vi "Measurement UI.vi"() -> ()   [LabVIEW 2025, in "Example Plugin UI.lvlib"]
uses:
  Example Plugin UI.lvlib
  ExamplePluginOOBService_client/RPC Messages/hwval_BoolRequest.ctl
  ExamplePluginOOBService_client/RPC Messages/hwval_ExportRequest.ctl
  ExamplePluginOOBService_client/ExamplePluginOOBService_client.lvlib
panel:
  out "Export out":string
  out "PauseResume out":bool
  in  "Export File Type":string(combo)="RAW"
  in  "Export":bool
  in  "PauseResume":bool caption="Pause"
  out "OOB Port":i32
  out "string 2D array out":string[][](array[string])
  in  "string 2D array in":string[][](array[string])
  out "double 2D array out":dbl[][](array[numeric])
  in  "double 2D array in":dbl[][](array[numeric])
  out "xy data out":cluster{"x_data":dbl[], "y_data":dbl[]}(graph)
  out "u32 animal enum out":enum32{"Rabbit", "Gopher", "Badger"}(ring)=enum."Badger"
  out "u32 color ring out":u32(ring)=2 items=["Red", "Green", "Blue"]
  out "string out":string="Empty"
  out "bool out":bool
  out "I64 out":i64
  out "I64 array out":i64[](array[numeric])
  out "I32 out":i32
  out "I32 array out":i32[](array[numeric])
  out "U64 out":u64
  out "U64 array out":u64[](array[numeric])
  out "U32 out":u32
  out "U32 array out":u32[](array[numeric])
  out "double out":dbl
  out "double array out":dbl[](array[numeric])
  in  "u32 animal enum in":enum32{"Rabbit", "Gopher", "Badger"}(ring)
  in  "u32 color ring in":u32(ring) items=["Red", "Green", "Blue"]
  in  "string in":string
  in  "bool in":bool
  in  "I64 in":i64
  in  "I64 array in":i64[](array[numeric])
  in  "I32 in":i32
  in  "I32 array in":i32[](array[numeric])
  in  "U64 in":u64
  in  "U64 array in":u64[](array[numeric])
  in  "U32 in":u32
  in  "U32 array in":u32[](array[numeric])
  in  "double in":dbl
  in  "double array in":dbl[](array[numeric])
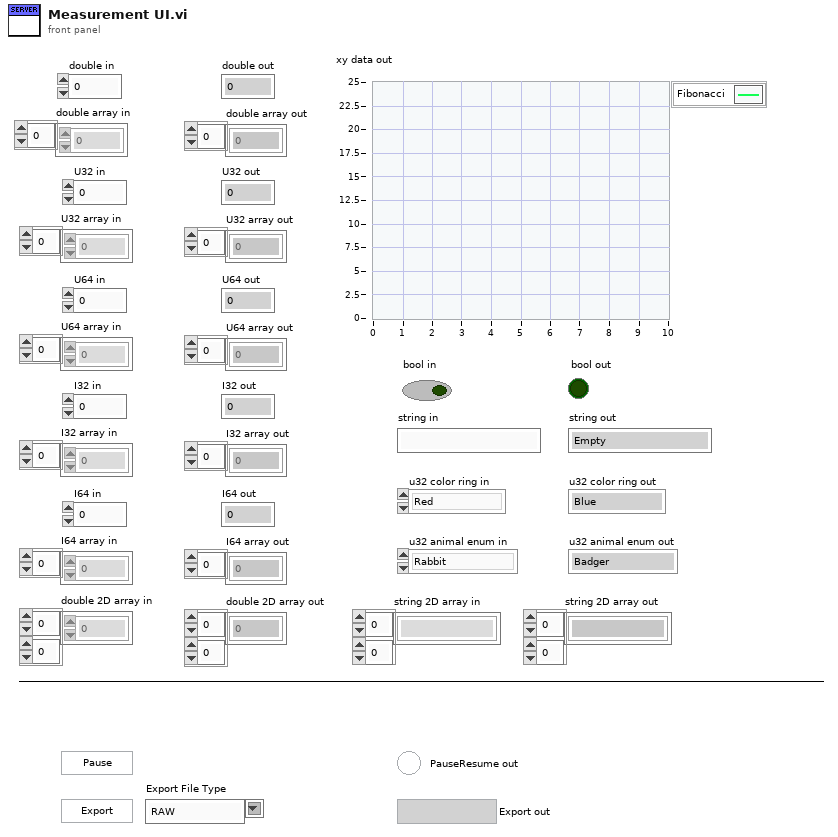
[diagram p1: front panel]
types:
  T1 = typedef "grpc-lvsupport-release.lvlib/grpcId.ctl" = u64
  T2 = typedef "ExamplePluginOOBService_client.lvlib/hwval_BoolRequest.ctl" = cluster{"BooleanData":bool}
  T3 = typedef "ExamplePluginOOBService_client.lvlib/hwval_ExportRequest.ctl" = cluster{"FileType":string}
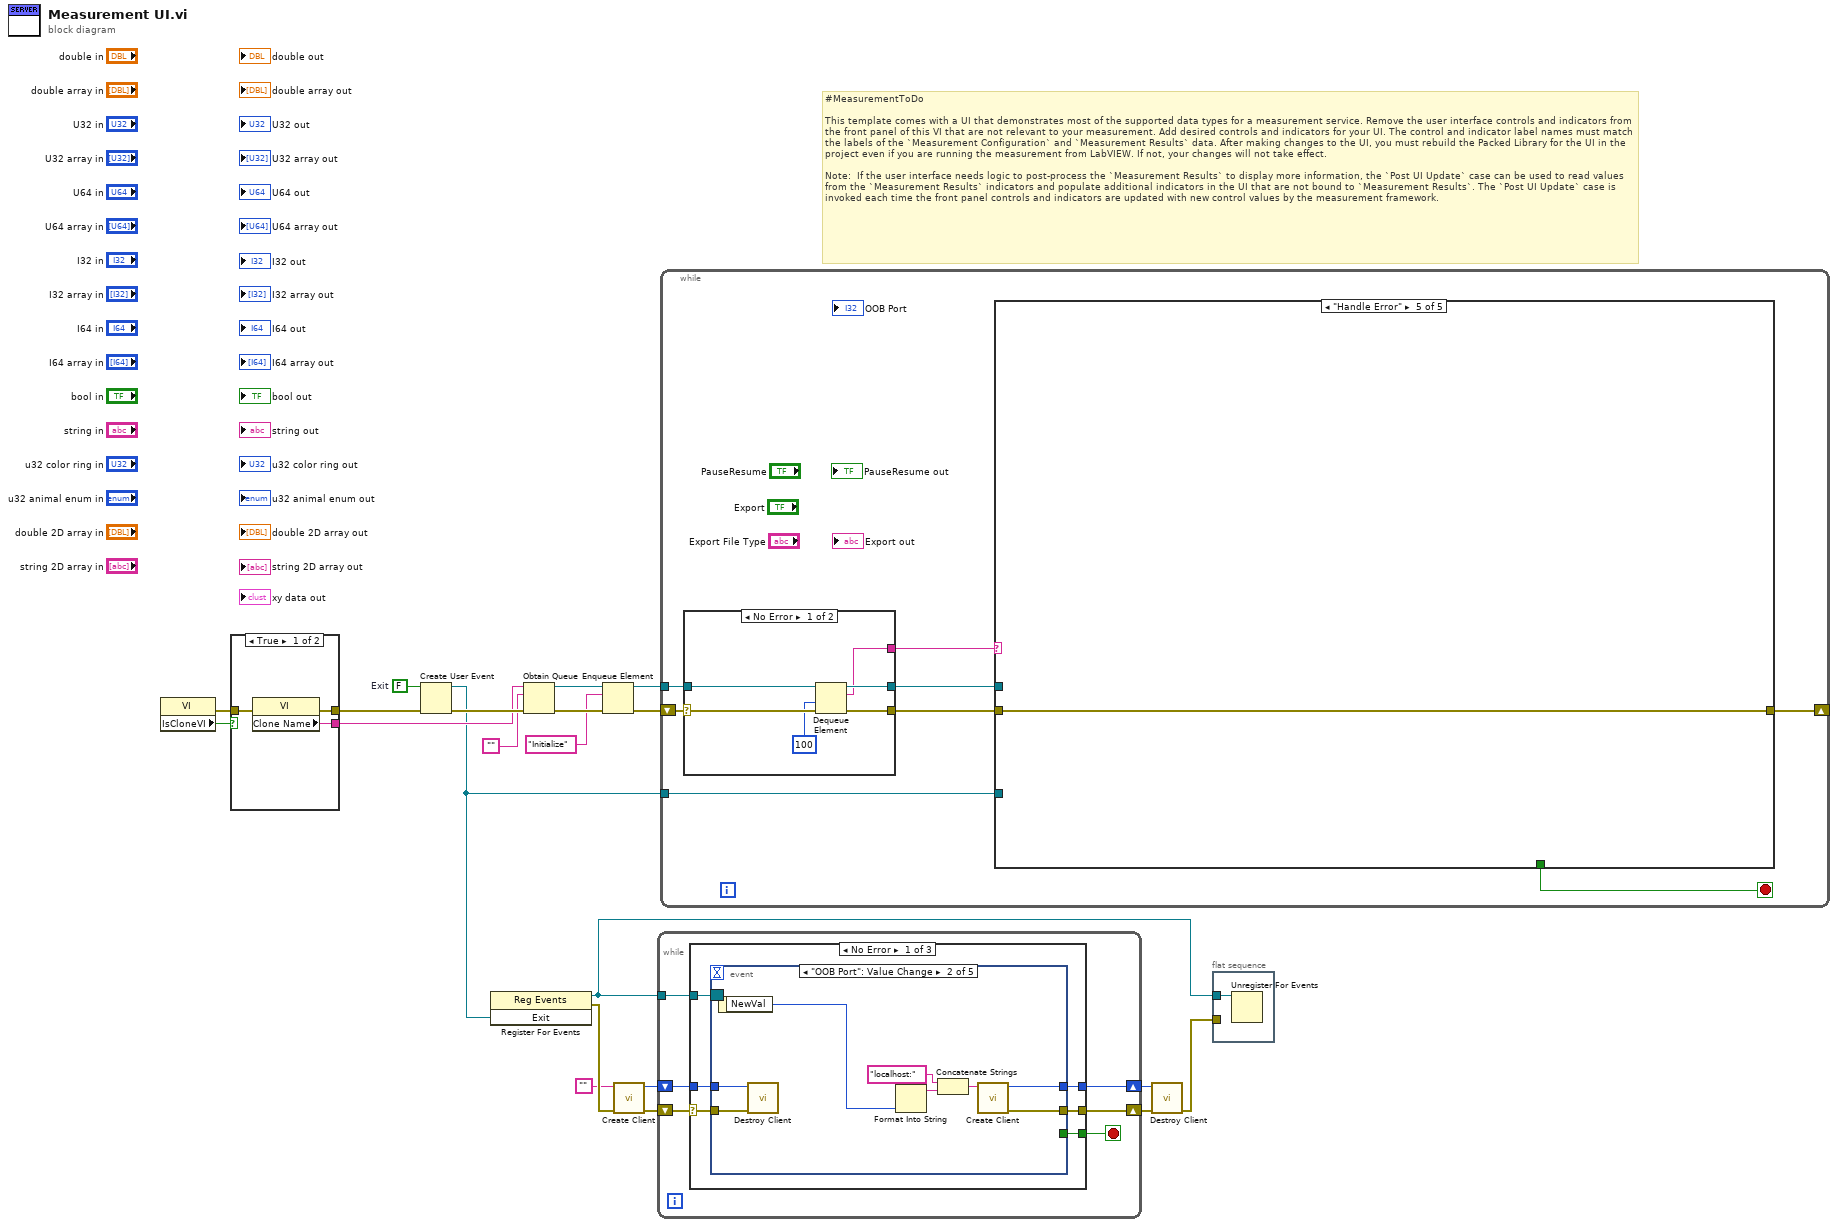
[diagram p0: block diagram]
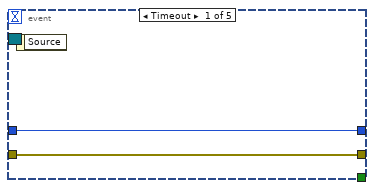
[diagram p2: hidden frame]
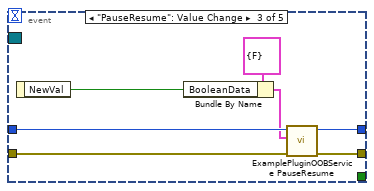
[diagram p3: hidden frame]
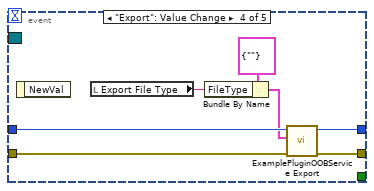
[diagram p4: hidden frame]
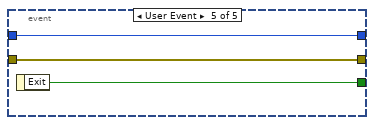
[diagram p5: hidden frame]
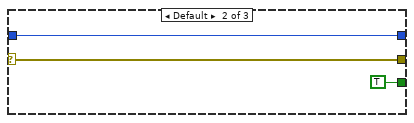
[diagram p6: hidden frame]
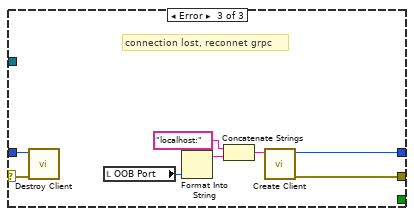
[diagram p7: hidden frame]
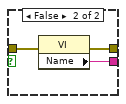
[diagram p8: hidden frame]
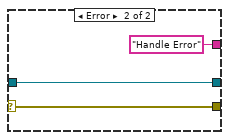
[diagram p9: hidden frame]
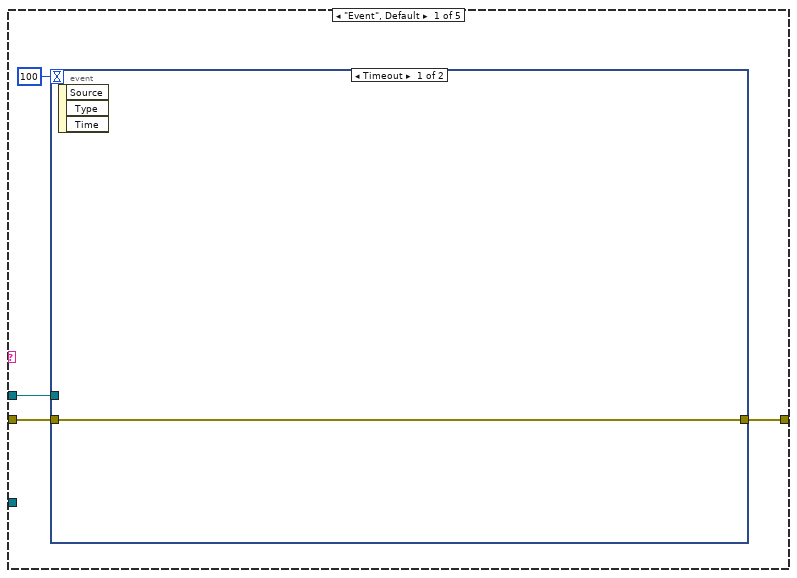
[diagram p10: hidden frame]
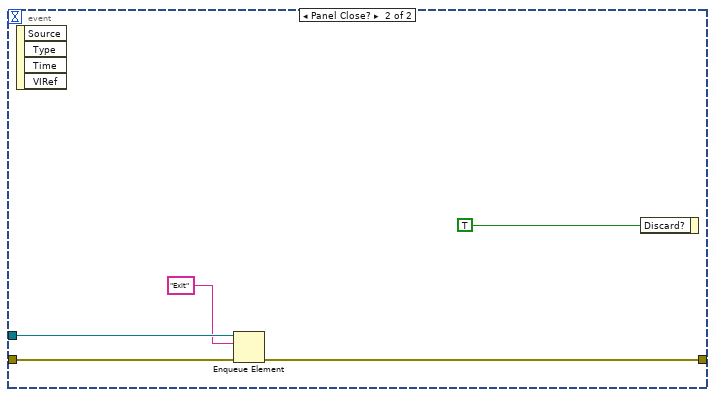
[diagram p11: hidden frame]
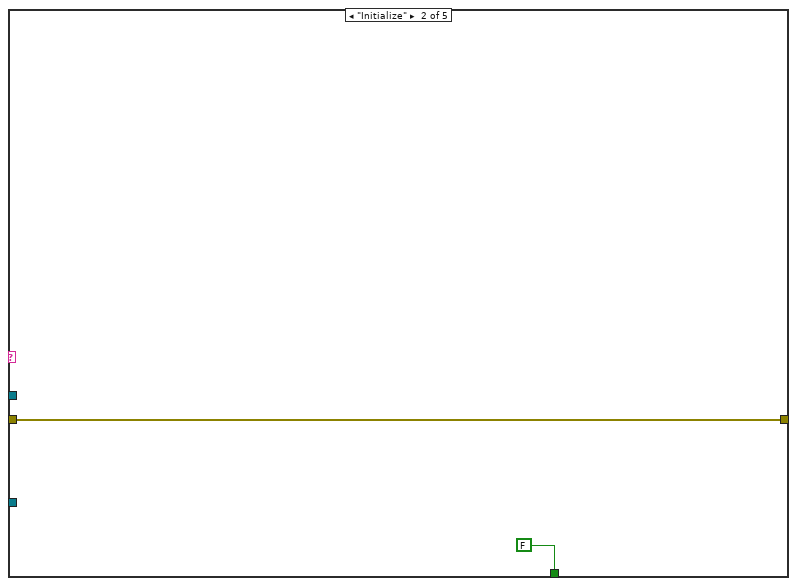
[diagram p12: hidden frame]
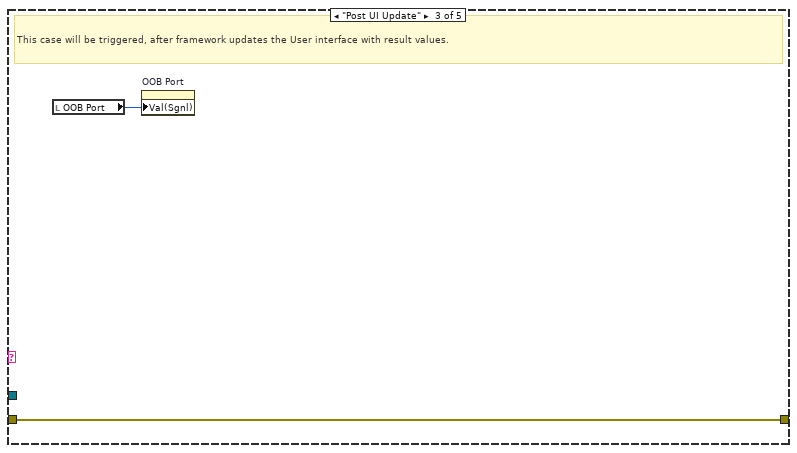
[diagram p13: hidden frame]
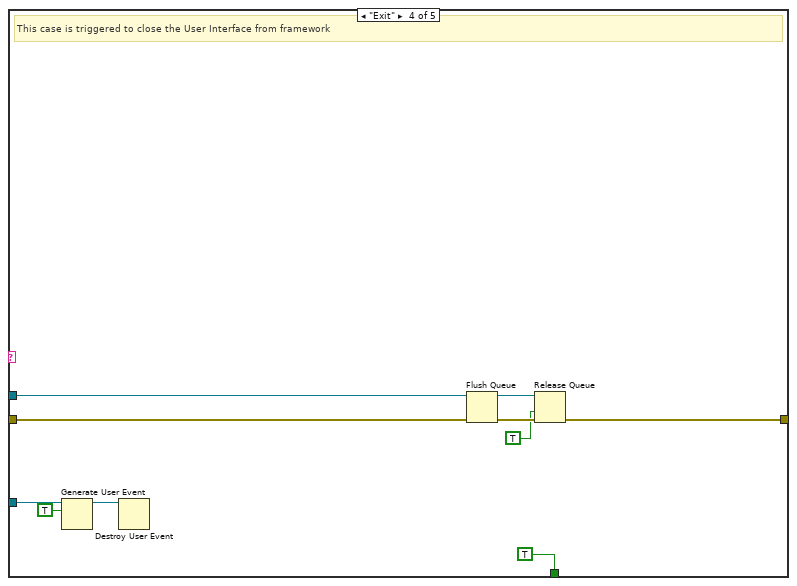
[diagram p14: hidden frame]
diagram:
  w11 = FALSE  # Exit
  # "#MeasurementToDo  \n\nThis template comes with a UI that demonstrates most of the supported data types for a measurement service. Remove the user interface controls and indicators from the front panel of this VI that are not relevant to your measurement. Add desired controls and indicators for your UI. The control and indicator label names must match the labels of the `Measurement Configuration` and `Measurement Results` data. After making changes to the UI, you must rebuild the Packed Library for the UI in the project even if you are running the measurement from LabVIEW. If not, your changes will not take effect.\n\nNote:  If the user interface needs logic to post-process the `Measurement Results` to display more information, the `Post UI Update` case can be used to read values from the `Measurement Results` indicators and populate additional indicators in the UI that are not bound to `Measurement Results`. The `Post UI Update` case is invoked each time the front panel controls and indicators are updated with new control values by the measurement framework."
  n1 = property class="VI"() -> (error out=w12:errorcluster, "IsCloneVI"=w13:bool)  [unwired: 2 in, 1 out]
  n2 = case shown="True" w13 {
    tunnel: [w24 w27] -> w10
    tunnel: [w23 w26] -> w20
    tunnel: w12 -> [w22 w25]
    frame True {
      n3 = property class="VI"(error in=w22) -> (error out=w24:errorcluster, "Clone Name"=w23:string)  [unwired: 1 in, 1 out]
    }
    frame False {
      n4 = property class="VI"(error in=w25) -> (error out=w27:errorcluster, "Name"=w26:string)  [unwired: 1 in, 1 out]
    }
  }
  n5 = Create User Event(user event datatype=w11, error in=w10) -> (user event=w3:refnum<user-event>, error out=w21:errorcluster)
  n6 = register-events(w3) -> (reference out=w9:refnum<event-registration>, error out=w8:errorcluster)  [unwired: 2 in]
  n7 = Obtain Queue(name (unnamed)=w20, element data type="", error in (no error)=w21) -> (queue out=w17:refnum<queue>, error out=w19:errorcluster)  [unwired: 2 in, 1 out]
  n8 = Enqueue Element(queue=w17, element="Initialize", error in (no error)=w19) -> (queue out=w16:refnum<queue>, error out=w18:errorcluster)  [unwired: 1 in, 1 out]
  n9 = call "Create Client.vi"("error in"=w8, "address"="") -> ("error out"=w1:errorcluster, "gRPC ID Out"=w2:T1)  [unwired: 8 in]
  n10 = while {
    tunnel: w9 -> [w30]
    shift-right: [w31] -> w6
    shift-left: w1 -> [w33]
    shift-right: [w28] -> w4
    shift-left: w2 -> [w29]
    stop <- w32 stop-if-true
    n11 = case shown="No Error" w33 {
      selector: w33 -> [w37 w68 w75]
      tunnel: [w34 TRUE _] -> w32
      tunnel: [w38 w68 w73] -> w31
      tunnel: w30 -> [w39 _ _]
      tunnel: w29 -> [w36 w67 w74]
      tunnel: [w35 w67 w72] -> w28
      frame No Error {
        n12 = event shown="[1] \"OOB Port\": Value Change" {
          selector: w39 -> [_ _ _ _ _]
          dyn-events: _ -> [_ _ _ _ _]
          timeout: _ -> [_ _ _ _ _]
          tunnel: [w41 w49 w55 w62 w64] -> w38
          tunnel: w37 -> [w41 w47 w53 w60 w64]
          tunnel: w36 -> [w40 w48 w54 w61 w65]
          tunnel: [w40 w42 w56 w63 w65] -> w35
          tunnel: [_ _ _ _ w66] -> w34
          event Timeout {
            n13 = event-data() -> ()  [unwired: 1 in, 1 out]
          }
          event "OOB Port": Value Change {
            n14 = event-data() -> ("NewVal"=w43:i32)  [unwired: 1 in]
            n15 = call "Destroy Client.vi"("error in"=w47, "gRPC ID"=w48) -> ()  [unwired: 9 in, 1 out]
            n16 = Format Into String(w43) -> (resulting string=w46:string)  [unwired: 3 in, 1 out]
            n17 = Concatenate Strings("localhost:" ("string"), w46) -> (w44:string)
            n18 = call "Create Client.vi"("address"=w44) -> ("error out"=w49:errorcluster, "gRPC ID Out"=w42:T1)  [unwired: 9 in]
          }
          event "PauseResume": Value Change {
            n19 = event-data() -> ("NewVal"=w50:bool)  [unwired: 1 in]
            n20 = Bundle By Name(cluster=T2 {"BooleanData"=FALSE} ("Request Data"), "BooleanData"=w50) -> (w51:T2)
            n21 = call "ExamplePluginOOBService PauseResume.vi"("error in"=w53, "Request Data"=w51, "gRPC ID"=w54) -> ("error out"=w55:errorcluster, "gRPC ID out"=w56:T1)  [unwired: 6 in, 1 out]
          }
          event "Export": Value Change {
            n22 = event-data() -> ()  [unwired: 1 in, 1 out]
            n23 = local read "Export File Type"() -> (w57:string)
            n24 = Bundle By Name(cluster=T3 {"FileType"=""} ("Request Data"), "FileType"=w57) -> (w58:T3)
            n25 = call "ExamplePluginOOBService Export.vi"("error in"=w60, "Request Data"=w58, "gRPC ID"=w61) -> ("error out"=w62:errorcluster, "gRPC ID out"=w63:T1)  [unwired: 6 in, 1 out]
          }
          event User Event {
            n26 = event-data() -> ("Exit"=w66:bool)  [unwired: 1 in]
          }
        }
      }
      frame Default {
      }
      frame Error {
        # "connection lost, reconnet grpc"
        n27 = call "Destroy Client.vi"("error in"=w75, "gRPC ID"=w74) -> ()  [unwired: 9 in, 1 out]
        n28 = local read "OOB Port"() -> (w71:i32)
        n29 = Format Into String(w71) -> (resulting string=w77:string)  [unwired: 3 in, 1 out]
        n30 = Concatenate Strings("localhost:" ("string"), w77) -> (w76:string)
        n31 = call "Create Client.vi"("address"=w76) -> ("error out"=w73:errorcluster, "gRPC ID Out"=w72:T1)  [unwired: 9 in]
      }
    }
  }
  n32 = while {
    shift-right: [w80] -> _
    shift-left: w18 -> [w85]
    tunnel: w16 -> [w83]
    tunnel: w3 -> [w78]
    stop <- w79 stop-if-true
    n33 = case shown="No Error" w85 {
      selector: w85 -> [w91 w94]
      tunnel: [w90 w94] -> w84
      tunnel: w83 -> [w89 w93]
      tunnel: [w88 w93] -> w82
      tunnel: [w87 "Handle Error"] -> w81
      frame No Error {
        n34 = Dequeue Element(queue=w89, timeout in ms (-1)=100, error in (no error)=w91) -> (queue out=w88:refnum<queue>, element=w87:string, error out=w90:errorcluster)  [unwired: 1 out]
      }
      frame Error {
      }
    }
    n35 = case shown="\"Handle Error\"" w81 {
      tunnel: w84 -> [w97 w106 w108 w118 w119]
      tunnel: w82 -> [w95 _ _ w116 _]
      tunnel: [w98 w106 w108 w113 w119] -> w80
      tunnel: [_ FALSE _ TRUE _] -> w79
      tunnel: w78 -> [_ _ _ w109 _]
      frame "Event", Default {
        n36 = event shown="[0] Timeout" {
          selector: _ -> [_ _]
          dyn-events: _ -> [_ _]
          timeout: 100 -> [_ _]
          tunnel: [w99 w102] -> w98
          tunnel: w97 -> [w99 w103]
          tunnel: w95 -> [_ w101]
          event Timeout {
            n37 = event-data() -> ()  [unwired: 1 in, 3 out]
          }
          event Panel Close? {
            n38 = event-data() -> ()  [unwired: 1 in, 4 out]
            n39 = Enqueue Element(queue=w101, element="Exit", error in (no error)=w103) -> (error out=w102:errorcluster)  [unwired: 1 in, 2 out]
            n40 = event-data("Discard?"=TRUE) -> ()  [unwired: 1 in, 1 out]
          }
        }
      }
      frame "Initialize" {
      }
      frame "Post UI Update" {
        # "This case will be triggered, after framework updates the User interface with result values."
        n41 = local read "OOB Port"() -> (w107:i32)
        n42 = property on="OOB Port" class="DigNum (strict)"("Val(Sgnl)"=w107) -> ()  [unwired: 2 in, 2 out]
      }
      frame "Exit" {
        # "This case is triggered to close the User Interface from framework"
        n43 = Generate User Event(user event=w109, event data cluster=TRUE ("event data")) -> (user event out=w110:refnum<user-event>)  [unwired: 2 in, 1 out]
        n44 = Destroy User Event(user event=w110) -> ()  [unwired: 1 in, 1 out]
        n45 = Flush Queue(queue=w116, error in (no error)=w118) -> (queue out=w115:refnum<queue>, error out=w114:errorcluster)  [unwired: 1 out]
        n46 = Release Queue(queue=w115, force destroy? (F)=TRUE, error in (no error)=w114) -> (error out=w113:errorcluster)  [unwired: 2 out]
      }
      frame "Handle Error" {
      }
    }
  }
  n47 = call "Destroy Client.vi"("error in"=w6, "gRPC ID"=w4) -> ("error out"=w5:errorcluster)  [unwired: 9 in]
  n48 = flat-sequence {
    tunnel: w9 -> [w120]
    tunnel: w5 -> [_]
    frame #0 {
      n49 = Unregister For Events(event registration refnum=w120) -> ()  [unwired: 1 in, 1 out]
    }
  }
